vi "Set Channel Group Channels.vi"(8 "error in":errorcluster, 9 "channels":T1[](array[typedef]) format="%.0x", 10 "names":string[](array[string]), 11 "channel group in":T1 format="%.0x") -> (0 "error out":errorcluster, 1 "saved channels":T1[](array[typedef]) format="%.0x", 2 "saved names":string[](array[string]), 3 "channel group out":T1 format="%.0x")   [LabVIEW 2027, in "Embedded Data Logger Scripting.lvlib"]
uses:
  Embedded Data Logger Scripting.lvlib
  <vilib>/NI VeriStand/Custom Device API/Custom Device Item Ref.ctl
  <vilib>/NI VeriStand/Custom Device API/Custom Device API.lvlib
  <vilib>/NI VeriStand/Custom Device Tools/Custom Device Utility Library/Custom Device Utility Library.lvlib
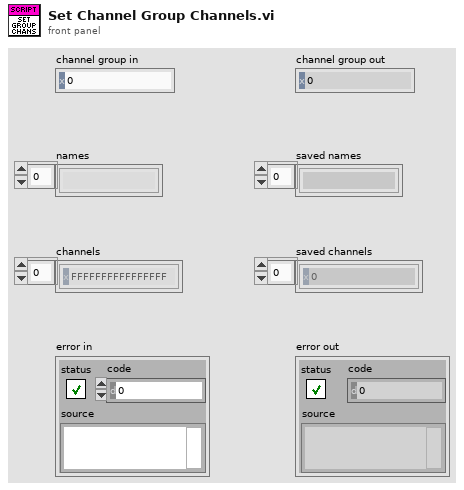
[diagram p1: front panel]
types:
  T1 = typedef "Custom Device API.lvlib/Custom Device Item Ref.ctl" = u64
  T2 = typedef "Custom Device API.lvlib/Custom Device Item Info.ctl" = cluster{"Name":string, "Is Channel":bool, "GUID":string, "Is Waveform":bool}
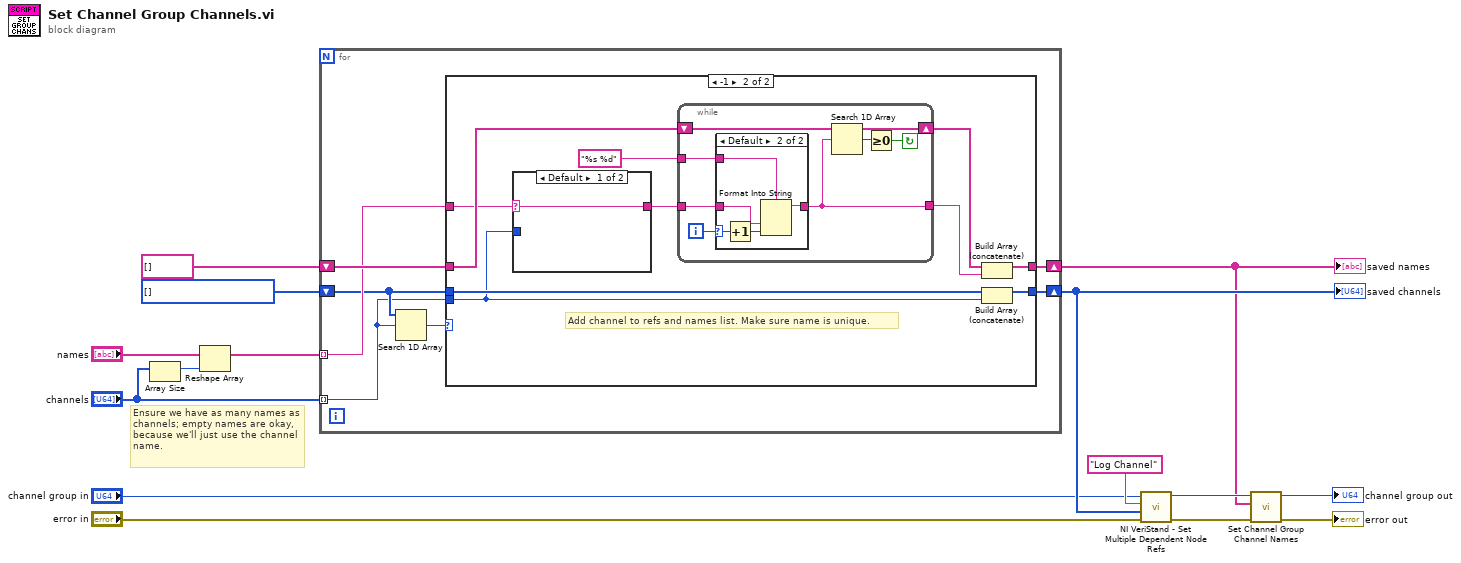
[diagram p0: block diagram]
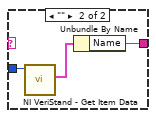
[diagram p3: hidden frame]
diagram:
  # "Ensure we have as many names as channels; empty names are okay, because we'll just use the channel name."
  n1 = Array Size(array="channels") -> (size(s)=w4:i32)
  n2 = Reshape Array("names", w4) -> (w5:string[])
  n3 = for {
    shift-right: [w22] -> w15
    shift-left: T1[] [] ("Selected Channel Refs") -> [w18]
    shift-right: [w20] -> w1
    shift-left: string[] [] -> [w21]
    tunnel: "channels" -> [w16] mode=indexing
    tunnel: w5 -> [w19] mode=indexing
    n4 = Search 1D Array(1D array=w18, element=w16) -> (index of element=w17:i32)  [unwired: 1 out]
    n5 = case shown="-1" w17 {
      tunnel: w18 -> [w24 w34]
      tunnel: [w24 w33] -> w22
      tunnel: w16 -> [_ w32]
      tunnel: w21 -> [w23 w28]
      tunnel: [w23 w31] -> w20
      tunnel: w19 -> [_ w25]
      frame Default {
        # "Channel already selected for logging. Don't add to refs or names list."
      }
      frame -1 {
        # "Add channel to refs and names list. Make sure name is unique."
        n6 = case shown="Default" w25 {
          selector: w25 -> [w35 _]
          tunnel: w32 -> [_ w38]
          tunnel: [w35 w36] -> w27
          frame Default {
          }
          frame "" {
            n7 = call <vilib>:"NI VeriStand - Get Item Data.vi"("Item Ref in"=w38) -> ("Item Info"=w37:T2)  [unwired: 1 in, 9 out]
            n8 = Unbundle By Name(w37) -> ("Name"=w36:string)
          }
        }
        n9 = while {
          shift-right: [w43] -> w29
          shift-left: w28 -> [w43]
          tunnel: w27 -> [w44]
          tunnel: [w40] -> w26
          tunnel: "%s %d" ("format string") -> [w39]
          i -> [w45]
          stop <- w41 continue-if-true
          n10 = case shown="Default" w45 {
            selector: w45 -> [_ w49]
            tunnel: w44 -> [w46 w47]
            tunnel: [w46 w51] -> w40
            tunnel: w39 -> [_ w50]
            frame 0 {
            }
            frame Default {
              n11 = Increment(x=w49) -> (x+1=w48:i32)
              n12 = Format Into String(format string=w50, w47, w48) -> (resulting string=w51:string)  [unwired: 2 in, 1 out]
            }
          }
          n13 = Search 1D Array(1D array=w43, element=w40) -> (index of element=w42:i32)  [unwired: 1 out]
          n14 = Greater Or Equal To 0?(x=w42) -> (x >= 0?=w41:bool)
        }
        n15 = Build Array (concatenate)(w29, w26) -> (w31:string[])
        n16 = Build Array (concatenate)(w34, w32) -> (w33:T1[])
      }
    }
  }
  "saved channels" <- w15
  "saved names" <- w1
  n17 = call <vilib>:"NI VeriStand - Set Multiple Dependent Node Refs.vi"("error in (no error)"="error in", "Dependent Node Refs"=w15, "Base Property Name"="Log Channel" ("Property Name"), "Item Ref in"="channel group in") -> ("error out"=w13:errorcluster, "Item Ref out"=w2:T1)  [unwired: 6 in]
  n18 = call "Set Channel Group Channel Names.vi"("error in (no error)"=w13, "names"=w1, "channel group in"=w2) -> ("error out"=→"error out":errorcluster, "channel group out"=→"channel group out":T1)  [unwired: 7 in]
